vi "Open plugin data.vi"(0 "Path":path, 11 "error in (no error)":errorcluster) -> (15 "error out":errorcluster)   [LabVIEW 2021, in "G Plug-in Migrator.lvlib"]
uses:
  G Plug-in Migrator.lvlib
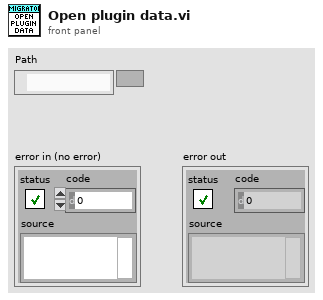
[diagram p1: front panel]
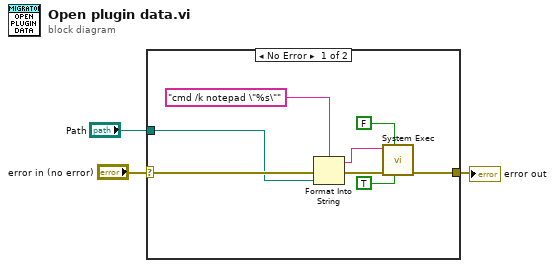
[diagram p0: block diagram]
diagram:
  n1 = case shown="No Error" "error in (no error)" {
    selector: "error in (no error)" -> [w6 w12]
    tunnel: [w4 w12] -> w3
    tunnel: "Path" -> [w5 _]
    frame No Error {
      n2 = Format Into String(format string="cmd /k notepad \"%s\"", error in=w6, w5) -> (resulting string=w8:string, error out=w11:errorcluster)  [unwired: 1 in]
      n3 = call <vilib>:"System Exec.vi"("run minimized? (F)"=TRUE, "wait until completion? (T)"=FALSE, "error in (no error)"=w11, "command line"=w8) -> ("error out"=w4:errorcluster)  [unwired: 4 in, 3 out]
    }
    frame Error {
    }
  }
  "error out" <- w3
